vi "Clear buffer.vi"(8 "error in (no error)":errorcluster, 11 "PS Driver AMI4xx in":refnum<class "PS Driver AMI4xx.lvclass">) -> (0 "error out":errorcluster, 3 "PS Driver AMI4xx out":refnum<class "PS Driver AMI4xx.lvclass">)   [LabVIEW 2022 SP3, in "PS Driver.lvlib" / "PS Driver AMI4xx.lvclass"]
uses:
  PS Driver AMI4xx.lvclass
  Y:/Winders LV 22/NML Data Acquisition/SCM PS Actor Framework/PS Driver/PS Driver.lvclass
  PS Driver.lvclass/PS Driver.ctl
  PS Driver.lvclass
panel:
  out "error out 2":errorcluster {"code" format="%.0x"}
  out "read buffer":string
  out "Timeout":u32
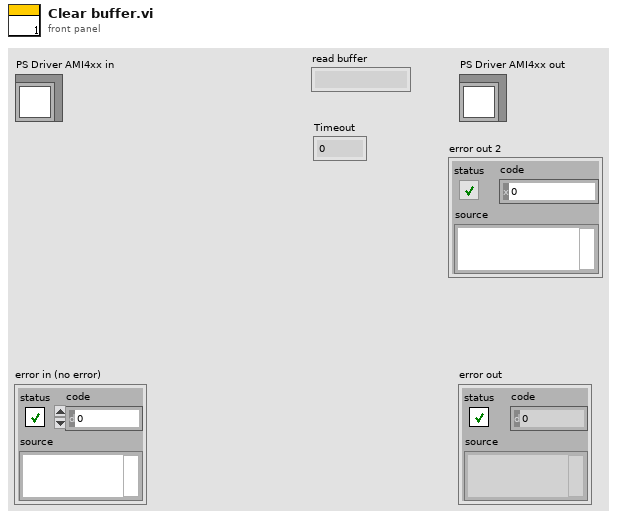
[diagram p1: front panel]
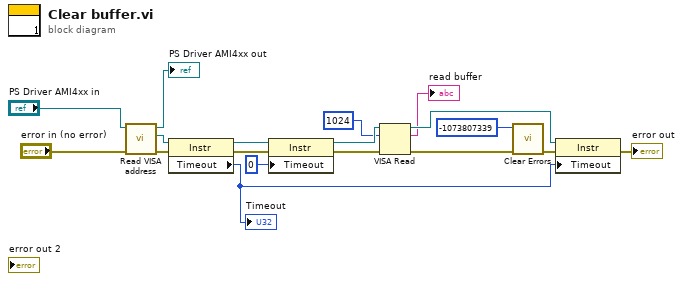
[diagram p0: block diagram]
diagram:
  n1 = call "Read VISA address.vi"("error in (no error)"="error in (no error)", "PS Driver in"="PS Driver AMI4xx in") -> ("error out"=w7:errorcluster, "VISA address"=w8:refnum<visa-resource-name>, "PS Driver out"=→"PS Driver AMI4xx out":refnum<class "PS Driver AMI4xx.lvclass">)  [unwired: 7 in]
  n2 = property class="Instr"(reference=w8, error in=w7) -> (reference out=w9:refnum<visa-resource-name>, error out=w6:errorcluster, "Timeout"=w4:u32)
  "Timeout" <- w4
  n3 = property class="Instr"(reference=w9, error in=w6, "Timeout"=u32 0 ("General Settings:Timeout Value")) -> (reference out=w15:refnum<visa-resource-name>, error out=w11:errorcluster)
  n4 = VISA Read(VISA resource name=w15, byte count=u32 1024, error in (no error)=w11) -> (VISA resource name out=w13:refnum<visa-resource-name>, read buffer=→"read buffer":string, error out=w2:errorcluster)  [unwired: 1 out]
  n5 = call <vilib>:"Clear Errors.vi"("error in (no error)"=w2, "specific error code to clear (0: all)"=-1073807339) -> ("error out"=w1:errorcluster)  [unwired: 4 in, 1 out]
  n6 = property class="Instr"(reference=w13, error in=w1, "Timeout"=w4) -> (error out=→"error out":errorcluster)  [unwired: 1 out]
